vi "S2DS_SETTINGS.vi"(0 "Instrument Info (out) in":T11, 1 "New sweep?":bool, 2 "Manual instruction?":bool, 3 "Script on?":bool, 5 "All channel parameters":T1 {"Scan parameters"."Y data taking" items=["in both direction", "in up direction only", "in down direction only"]; "Scan parameters"."X data taking" items=["in both direction", "in up direction only", "in down direction only"]}, 7 "External control settings":i32[](array[numeric]), 9 "Data save info (in)":T10={"File path"=path "", "Header"="", "File name"="", "False channel"=[], "Channel names"=[], "Buffer size"=0, "Format"="%.6f"}, 11 "error in (no error)":errorcluster, 12 "Prameter error":refnum<vi>, 13 "Script On?":refnum<vi>) -> (4 "Instrument Info (out) out":T11, 6 "All channel parameters (out)":T1 {"Scan parameters"."Y data taking" items=["in both direction", "in up direction only", "in down direction only"]; "Scan parameters"."X data taking" items=["in both direction", "in up direction only", "in down direction only"]}, 8 "Update instruction":i32[](array[numeric]), 10 "Data save info (out)":T10={"File path"=path "", "Header"="", "File name"="", "False channel"=[], "Channel names"=[], "Buffer size"=0, "Format"="%.6f"}, 14 "External control settings out":i32[](array[numeric]), 15 "error out":errorcluster)   [LabVIEW 2025]
uses:
  TYPE DEFS/S2DS_Instrument Info.ctl
  TYPE DEFS/S2DS_Instrument parameters.ctl
  TYPE DEFS/S2DS_Data saving info.ctl
  TYPE DEFS/S2DS_All Channel Parameters.ctl
  TYPE DEFS/S2DS_WC info.ctl
  TYPE DEFS/S2DS_Single WC info.ctl
  TYPE DEFS/S2DS_RC info.ctl
  TYPE DEFS/S2DS_Single RC info.ctl
  TYPE DEFS/S2DS_DAC info new.ctl
  TYPE DEFS/S2DS_Single DC info.ctl
  TYPE DEFS/S2DS_Array Inst Info.ctl
  TYPE DEFS/S2DS_Sweep Info.ctl
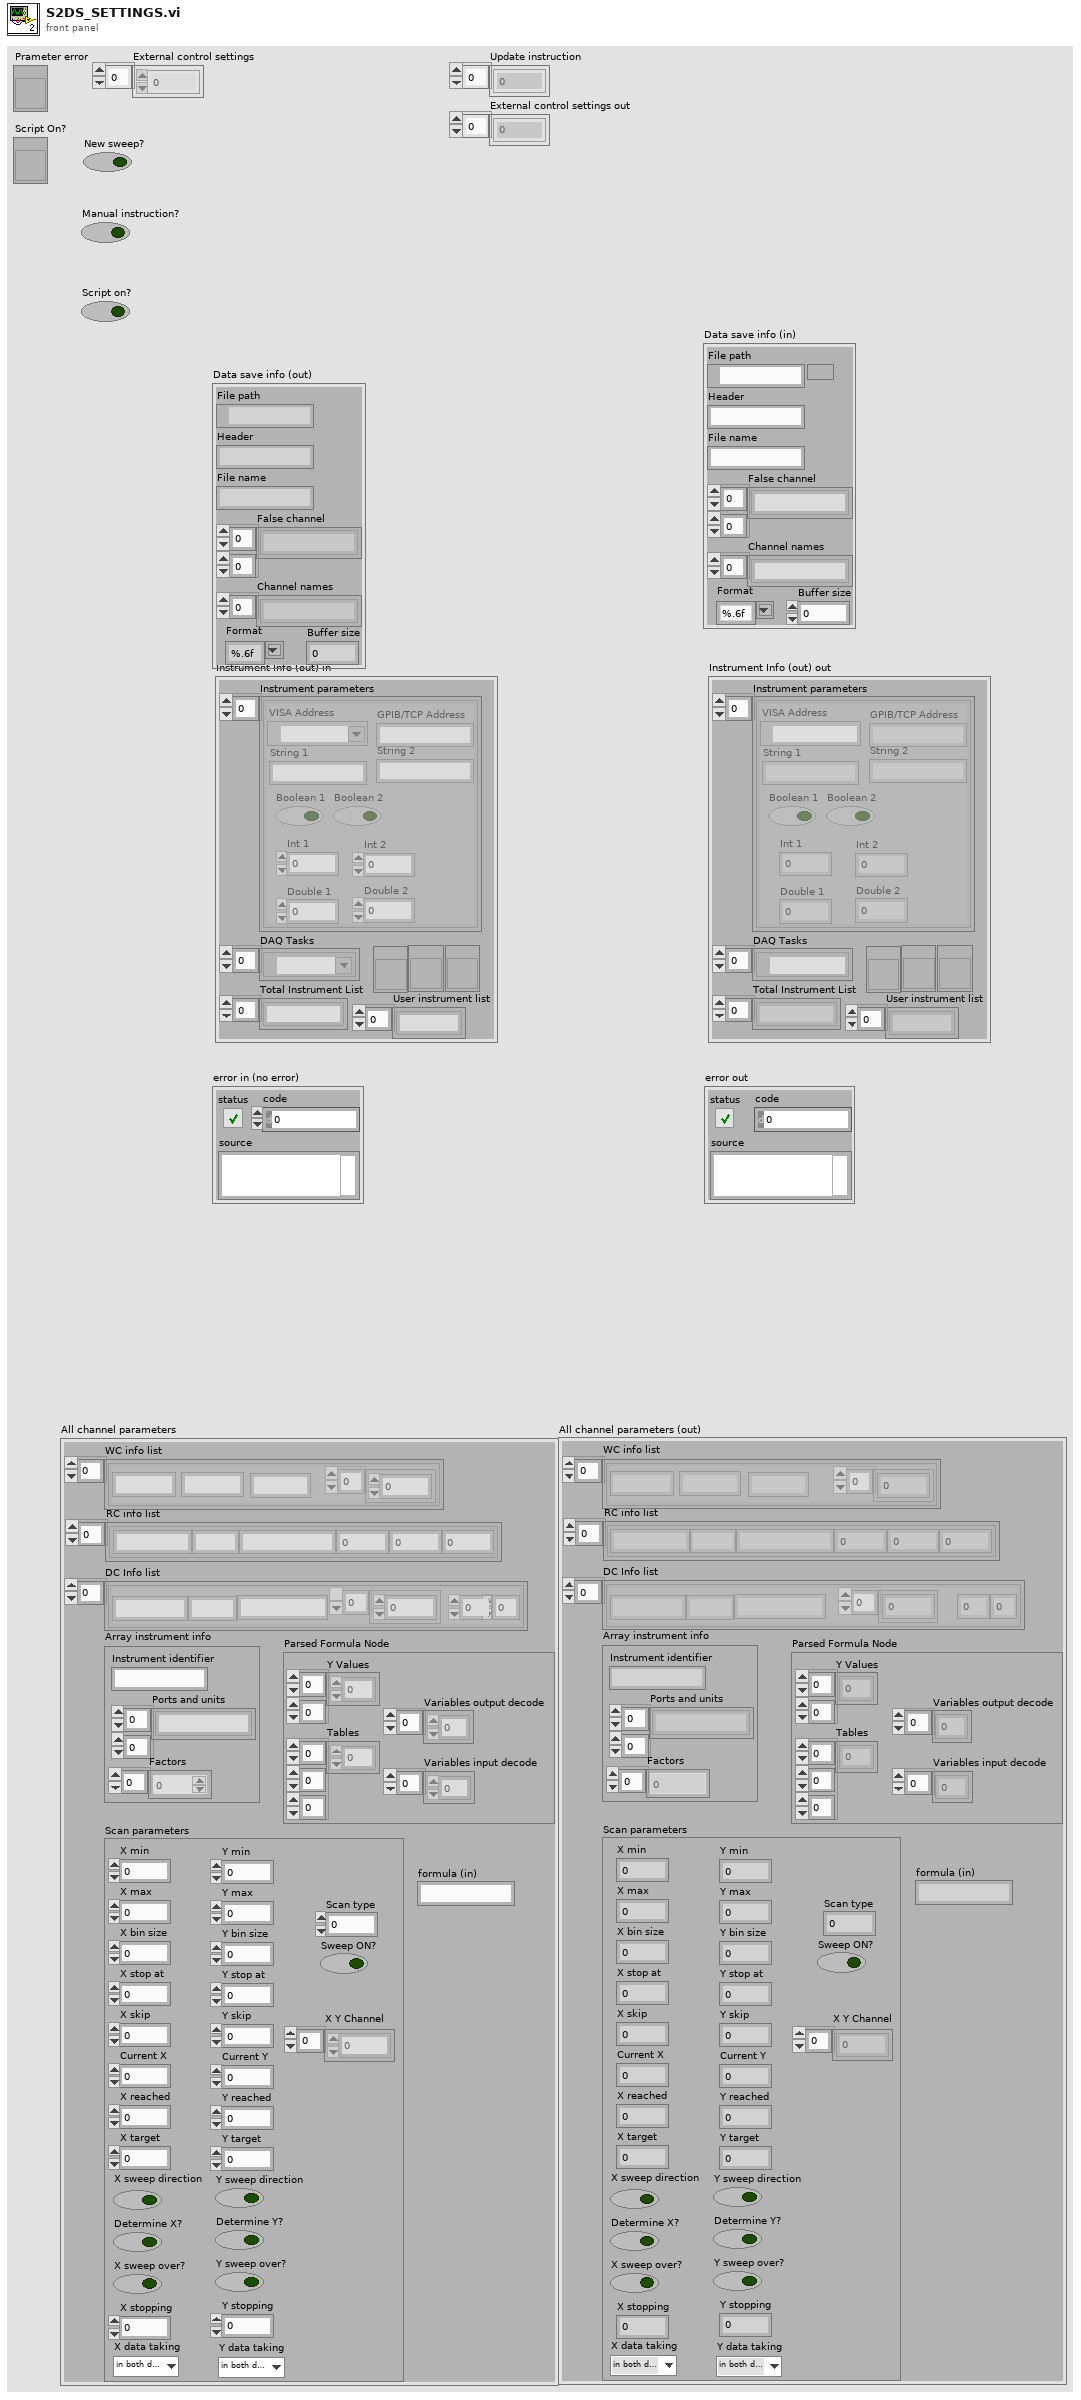
[diagram p1: front panel]
types:
  T1 = typedef "S2DS_All Channel Parameters.ctl" = cluster{"WC info list":T2, "RC info list":T4, "DC Info list":T6, "Array instrument info":T8, "Scan parameters":T9, "Parsed Formula Node":cluster{"Y Values":dbl[][], "Tables":i32[][][], "Variables input decode":i32[], "Variables output decode":i32[]}, "formula (in)":string}
  T2 = typedef "S2DS_WC info.ctl" = T3[]
  T3 = typedef "S2DS_Single WC info.ctl" = cluster{"Instrument identifier":string, "Write channel parameters":dbl[], "Name":string, "Unit":string}
  T4 = typedef "S2DS_RC info.ctl" = T5[]
  T5 = typedef "S2DS_Single RC info.ctl" = cluster{"Instrument identifier":string, "Factor":dbl, "Averaging":i32, "Wait (ms)":i32, "Unit":string, "Name":string}
  T6 = typedef "S2DS_DAC info new.ctl" = T7[]
  T7 = typedef "S2DS_Single DC info.ctl" = cluster{"Operation identifier":string, "DC parameters":dbl[], "U":i32, "V":i32, "Name":string, "Unit":string}
  T8 = typedef "S2DS_Array Inst Info.ctl" = cluster{"Instrument identifier":string, "Ports and units":string[][], "Factors":dbl[]}
  T9 = typedef "S2DS_Sweep Info.ctl" = cluster{"X min":ext, "X max":dbl, "Y min":dbl, "Y max":dbl, "X bin size":dbl, "Y bin size":dbl, "X stop at":dbl, "Y stop at":dbl, "X skip":u64, "Y skip":u64, "Current X":dbl, "Current Y":dbl, "X reached":i32, "Y reached":i32, "X target":dbl, "Y target":dbl, "Sweep ON?":bool, "X sweep direction":bool, "Y sweep direction":bool, "Determine X?":bool, "Determine Y?":bool, "X sweep over?":bool, "Y sweep over?":bool, "Scan type":i32, "X stopping":i32, "Y stopping":i32, "X Y Channel":u16[], "X data taking":u16, "Y data taking":u16}
  T10 = typedef "S2DS_Data saving info.ctl" = cluster{"File path":path, "Header":string, "File name":string, "False channel":string[][], "Channel names":string[], "Buffer size":i32, "Format":string}
  T11 = typedef "S2DS_Instrument Info.ctl" = cluster{"Instrument parameters":T12[], "DAQ Tasks":refnum<k21>[], "Total Instrument List":string[], "read inst \nVI Refnum":refnum<vi>, "type specifier Edit instruments VI Refnum":refnum<vi>, "type specifier write instrument VI Refnum (for type only)":refnum<vi>, "User instrument list":string[]}
  T12 = typedef "S2DS_Instrument parameters.ctl" = cluster{"VISA Address":refnum<visa-resource-name>, "GPIB/TCP Address":string, "String 1":string, "String 2":string, "Boolean 1":bool, "Boolean 2":bool, "Int 1":i32, "Int 2":i32, "Double 1":dbl, "Double 2":dbl}
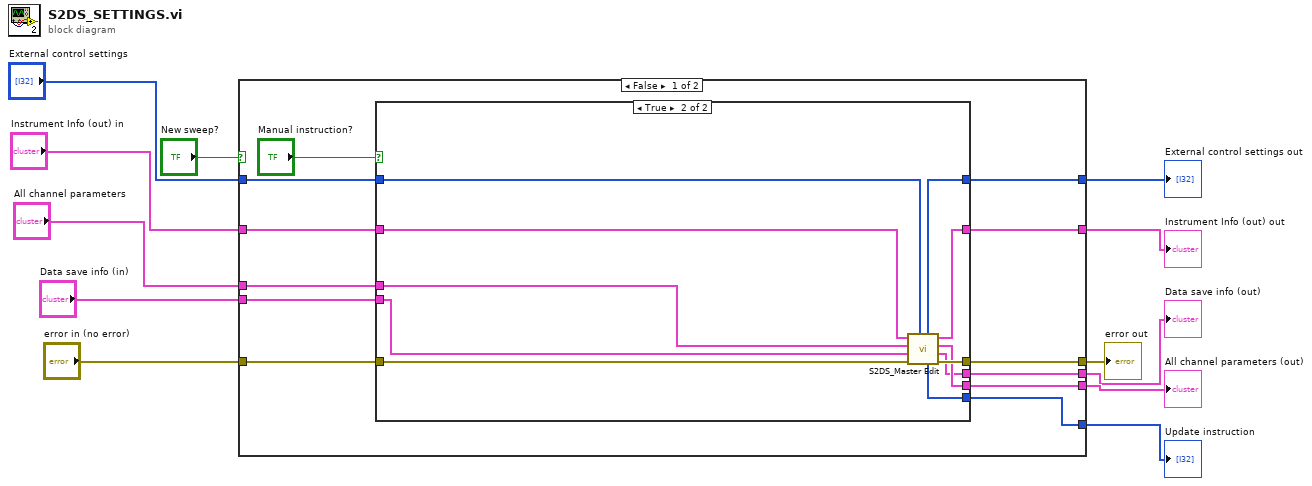
[diagram p0: block diagram]
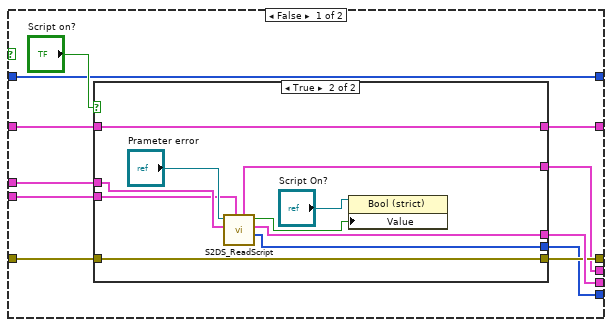
[diagram p2: hidden frame]
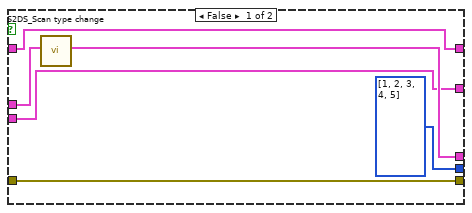
[diagram p3: hidden frame]
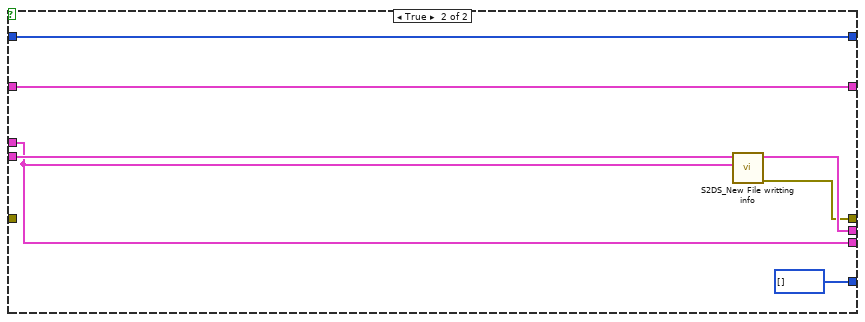
[diagram p4: hidden frame]
diagram:
  n1 = case shown="False" "New sweep?" {
    tunnel: "All channel parameters" -> [w24 w66]
    tunnel: "Data save info (in)" -> [w23 w67]
    tunnel: [w22 w69] -> w11
    tunnel: "Instrument Info (out) in" -> [w21 w69]
    tunnel: "error in (no error)" -> [w20 _]
    tunnel: [w19 w65] -> w5
    tunnel: [w17 w66] -> w8
    tunnel: [w16 w64] -> w7
    tunnel: [w15 i32[] [] ("Update instruction")] -> w6
    tunnel: "External control settings" -> [w14 w63]
    tunnel: [w13 w63] -> w2
    frame False {
      n2 = case shown="True" "Manual instruction?" {
        tunnel: w24 -> [w35 w61]
        tunnel: w23 -> [w26 w55]
        tunnel: [w25 w54] -> w19
        tunnel: [w34 w57] -> w17
        tunnel: [w33 w58] -> w22
        tunnel: [w32 w59] -> w16
        tunnel: w20 -> [w31 w60]
        tunnel: w21 -> [w30 w62]
        tunnel: [w29 w56] -> w15
        tunnel: w14 -> [w27 w53]
        tunnel: [w27 w52] -> w13
        frame False {
          n3 = case shown="True" "Script on?" {
            tunnel: w35 -> [w38 w47]
            tunnel: [w37 w46] -> w34
            tunnel: [w41 w51] -> w33
            tunnel: [w40 w50] -> w32
            tunnel: w31 -> [w40 w50]
            tunnel: w30 -> [w41 w51]
            tunnel: [i32[] [1, 2, 3, 4, 5] ("update instruction") w48] -> w29
            tunnel: w26 -> [w36 w43]
            tunnel: [w36 w42] -> w25
            frame False {
              n4 = call "S2DS_Scan type change.vi"("All channel parameters"=w38) -> ("All channel parameters (out)"=w37:T1)  [unwired: 10 in]
            }
            frame True {
              n5 = call "S2DS_ReadScript.vi"("Data save info (in)"=w43, "All channel parameters"=w47, "Status"="Prameter error") -> ("update instruction"=w48:i32[], "All channel parameters (out)"=w46:T1, "Script complete?"=w44:bool, "Data save info (out)"=w42:T10)  [unwired: 4 in, 1 out]
              n6 = property on="Property Node" class="Bool (strict)"(reference="Script On?", "Value"=w44) -> ()  [unwired: 1 in, 2 out]
            }
          }
        }
        frame True {
          n7 = call "S2DS_Master Edit.vi"("External control settings"=w53, "error in"=w60, "Data saving info"=w55, "All channel parameters"=w61, "Instrument Info (in)"=w62) -> ("error out"=w59:errorcluster, "Data saving info (out)"=w54:T10, "All channel parameters (out)"=w57:T1, "Instrument Info (out)"=w58:T11, "Update instruction"=w56:i32[], "External control settings out"=w52:i32[])  [unwired: 1 in]
        }
      }
    }
    frame True {
      n8 = call "S2DS_New File writting info.vi"("All channel parameters"=w66, "File info (in)"=w67) -> ("error out"=w64:errorcluster, "File info (out)"=w65:T10)  [unwired: 8 in]
    }
  }
  "Data save info (out)" <- w5
  "All channel parameters (out)" <- w8
  "Instrument Info (out) out" <- w11
  "error out" <- w7
  "Update instruction" <- w6
  "External control settings out" <- w2
